vi "initialaize.vi"(8 "error in (no error)":errorcluster, 9 "Visa com port":refnum<visa-resource-name>, 10 "Serial Device Brand":T1, 11 "Simulado in":refnum<class "Simulado.lvclass">) -> (0 "error out":errorcluster, 3 "Simulado out":refnum<class "Simulado.lvclass">)   [LabVIEW 2020, in "Simulado.lvclass"]
uses:
  Simulado.lvclass
  Combo box/serial device brand.ctl
  Abstracts/Serial Device/Serial Device.lvclass
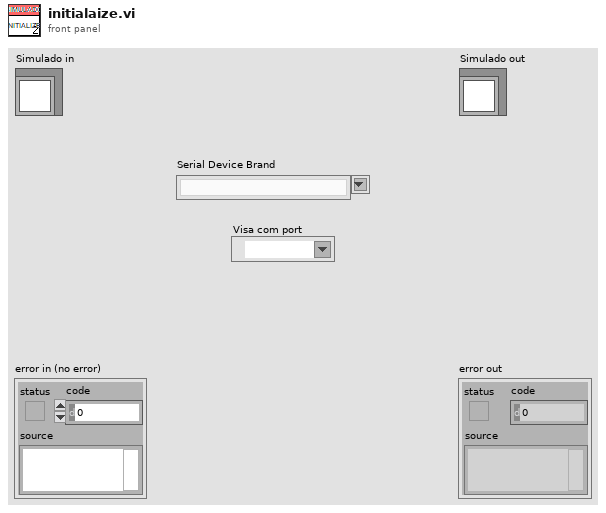
[diagram p1: front panel]
types:
  T1 = typedef "Serial Device.lvclass/serial device brand.ctl" = string
  T2 = enum16{"reset parameters", "Get parameters", "Set parameter"}
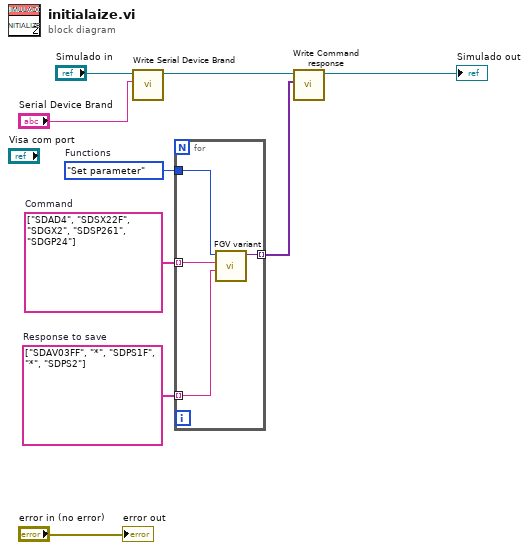
[diagram p0: block diagram]
diagram:
  w7 = string[] ["SDAV03FF", "*", "SDPS1F", "*", "SDPS2"]  # Response to save
  w8 = string[] ["SDAD4", "SDSX22F", "SDGX2", "SDSP261", "SDGP24"]  # Command
  w9 = T2."Set parameter"  # Functions
  n1 = call-dynamic "Write Serial Device Brand.vi"("Serial Device Brand"="Serial Device Brand", "Serial Device in"="Simulado in") -> ("Serial Device out"=w6:refnum<class "Simulado.lvclass">)  [unwired: 8 in, 1 out]
  n2 = for {
    tunnel: w9 -> [w13]
    tunnel: w8 -> [w12] mode=indexing
    tunnel: w7 -> [w11] mode=indexing
    tunnel: [w10] -> w3 mode=indexing
    n3 = call "FGV variant.vi"("Response to save"=w11, "Command"=w12, "Functions"=w13) -> ("Variant"=w10:variant)  [unwired: 7 in, 1 out]
  }
  n4 = call-dynamic "Write Command response.vi"("Command response"=w3, "Simulado in"=w6) -> ("Simulado out"=→"Simulado out":refnum<class "Simulado.lvclass">)  [unwired: 8 in, 1 out]
  "error out" <- "error in (no error)"
